vi "set temperature SINEWAVE - V1.vi"(10 "sweep folder path":path, 11 "Set Temperature PID":T1) -> (0 "next set temperature":dbl, 1 "set temperature points":dbl[](array[numeric]), 2 "time points (min)":dbl[](array[numeric]), 3 "Set Temperature PID OUT":T1)   [LabVIEW 2015]
uses:
  Set Temperature PID - Control.ctl
  next chunk read-write PID -- action.ctl
  ctl -- name dispatcher -- action.ctl
  file -- 9w path.vi
  array -- find index - real.vi
  array -- interpolate -- i.vi
  ctl -- name dispatcher.vi
  Q -- check range -- i -- real.vi
  Q - not nan -- real.vi
  <vilib>/Utility/libraryn.llb/Check if File or Folder Exists.vi
  file -- read list of lines.vi
  parse -- find first line.vi
  parse -- get list of matches -- numbers.vi
  <vilib>/Utility/file.llb/Write To Spreadsheet File.vi
  <vilib>/Utility/file.llb/Write To Spreadsheet File (string).vi
  <vilib>/gmath/function.llb/Binomial Coefficient.vi
panel:
  out "time(min)":dbl
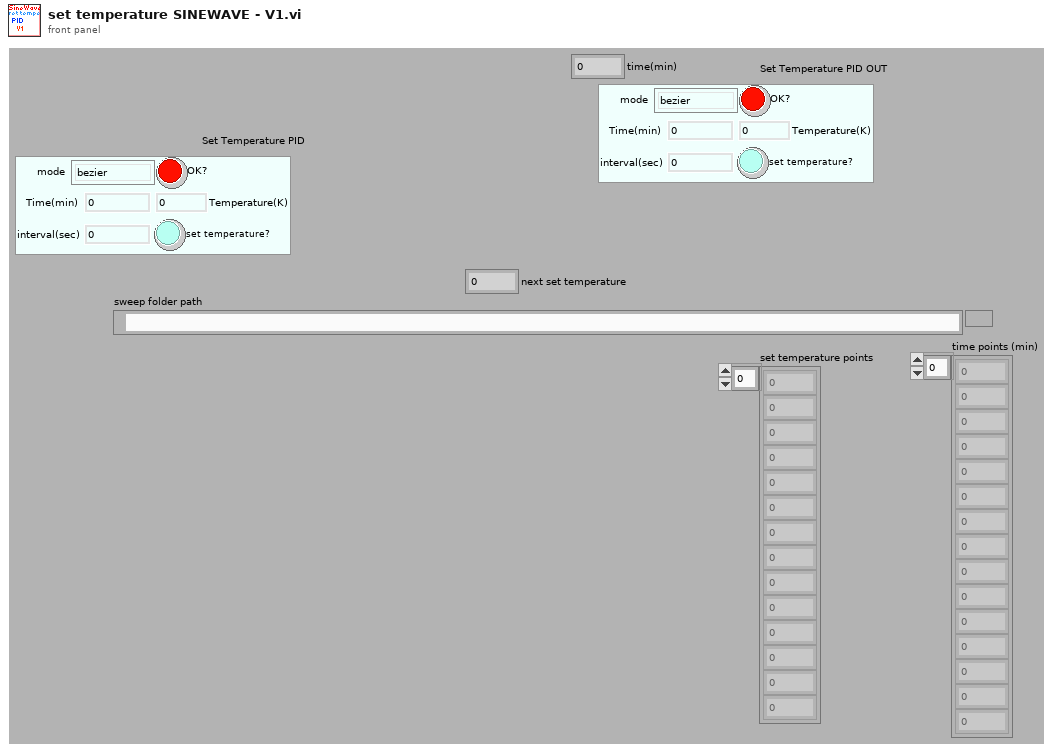
[diagram p1: front panel]
types:
  T1 = typedef "Set Temperature PID - Control.ctl" = cluster{"mode ":enum16{"bezier", "sine wave"}, "set temperature?":bool, "Time(min)":dbl, "Temperature(K)":dbl, "OK?":bool, "interval(sec)":dbl}
  T2 = typedef "next chunk read-write PID -- action.ctl" = enum16{"read", "interpolate", "append col", "write", "write PID col", "append PID col", "interpolate - bezier"}
  T3 = typedef "ctl -- name dispatcher -- action.ctl" = enum16{"peak frequency", "peak frequency DUMP", "peak gamma DUMP", "peak gamma", "peak frequency TEST", "peak gamma TEST", "ultrasonic power", "time in gamma", "set temperature ", "set temperature timer", "peak default gamma", "last scan file", "peak freq gamma TEST", "peak NAMES", "errors", "P_I_D", "P", "I", "D", "power vs time", "power vs time TIMER", "void", "power log", "set temperature - SINE", "itc ltc log", "peak - time in gamma"}
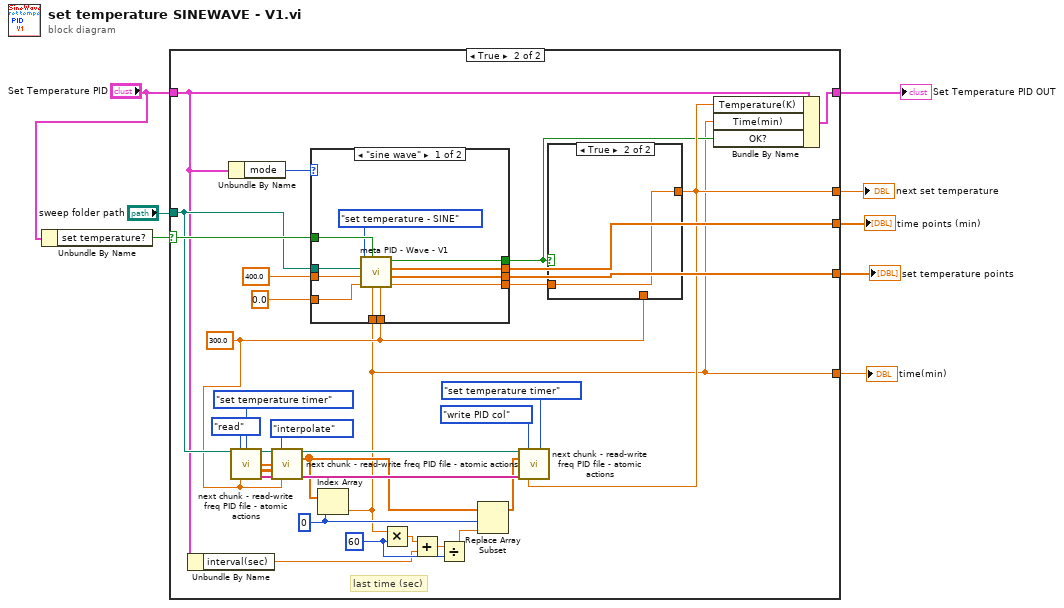
[diagram p0: block diagram]
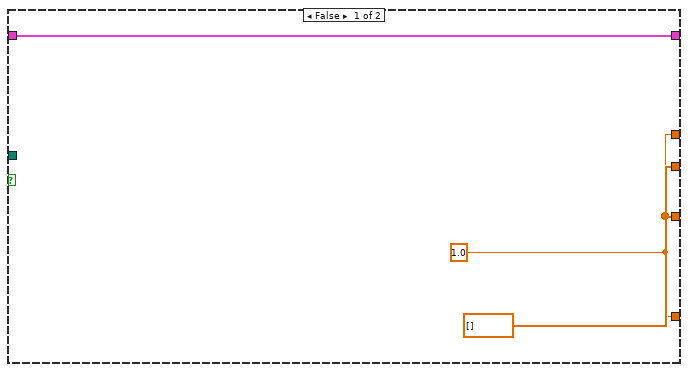
[diagram p2: hidden frame]
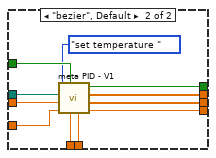
[diagram p3: hidden frame]
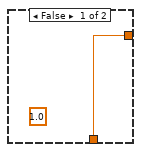
[diagram p4: hidden frame]
diagram:
  n1 = Unbundle By Name("Set Temperature PID") -> ("set temperature?"=w1:bool)
  n2 = case shown="True" w1 {
    selector: w1 -> [_ w41]
    tunnel: "sweep folder path" -> [_ w36]
    tunnel: [w10 w17] -> w7
    tunnel: [w11 w39] -> w6
    tunnel: [w11 w40] -> w5
    tunnel: [w10 w15] -> w4
    tunnel: "Set Temperature PID" -> [w9 w13]
    tunnel: [w9 w14] -> w3
    frame False {
      w11 = dbl[] [] ("temperatures")
      w10 = 1.0 ("upper")
    }
    frame True {
      w19 = 300.0 ("temperature")
      w27 = 0 ("index")
      w22 = 60
      # "last time (sec)"
      n3 = Unbundle By Name(w13) -> ("interval(sec)"=w12:dbl)
      n4 = Unbundle By Name(w13) -> ("mode"=w18:enum16{"bezier", "sine wave"})
      n5 = call "next chunk - read-write freq PID file - atomic actions .vi"("sweep folder path"=w36, "PID action"=next_chunk_read-write_PID_--_action."read", "ctl kind IN"=ctl_--_name_dispatcher_--_action."set temperature timer", "temperature"=w19) -> ("sweep folder path out"=w35:path, "temperatures"=w31:dbl[], "frequencies"=w30:dbl[][], "header"=w32:string[])  [unwired: 7 in, 1 out]
      n6 = call "next chunk - read-write freq PID file - atomic actions .vi"("PID action"=next_chunk_read-write_PID_--_action."interpolate", "temperatures IN"=w31, "frequencies IN"=w30, "header IN"=w32, "temperature"=w19) -> ("PID freq"=w23:dbl[], "header"=w28:string[])  [unwired: 6 in, 3 out]
      n7 = Index Array(array=w23, index=w27) -> (element=w15:dbl)
      n8 = case shown="\"sine wave\"" w18 {
        tunnel: 0.0 ("lower") -> [w54 w65]
        tunnel: 400.0 ("upper") -> [w53 w64]
        tunnel: w41 -> [w52 w63]
        tunnel: [w51 w62] -> w40
        tunnel: [w50 w61] -> w39
        tunnel: [w49 w60] -> w16
        tunnel: w36 -> [w48 w59]
        tunnel: [w47 w58] -> w20
        tunnel: w19 -> [w45 w56]
        tunnel: w15 -> [w44 w55]
        frame "sine wave" {
          n9 = call "meta PID - Wave - V1.vi"("default output"=w45, "input parameter"=w44, "control?"=w52, "lower limit"=w54, "upper limit"=w53, "sweep folder path"=w48, "ctl name dispatch"=ctl_--_name_dispatcher_--_action."set temperature - SINE") -> ("output"=w47:dbl, "frequencies"=w51:dbl[], "temperatures"=w50:dbl[], "ok"=w49:bool)  [unwired: 1 in]
        }
        frame "bezier", Default {
          n10 = call "meta PID - V1.vi"("default output"=w56, "input parameter"=w55, "control?"=w63, "lower limit"=w65, "upper limit"=w64, "sweep folder path"=w59, "ctl name dispatch"=ctl_--_name_dispatcher_--_action."set temperature ") -> ("bezier output"=w58:dbl, "frequencies"=w62:dbl[], "temperatures"=w61:dbl[], "ok"=w60:bool)  [unwired: 1 in]
        }
      }
      n11 = Multiply(x=w15, y=w22) -> (x*y=w21:dbl)
      n12 = Add(x=w21, y=w12) -> (x+y=w25:dbl)
      n13 = Divide(x=w25, y=w22) -> (x/y=w24:dbl)
      n14 = Replace Array Subset(array=w23, new element=w24, index=w27) -> (w26:dbl[])
      n15 = case shown="True" w16 {
        tunnel: [w66 w67] -> w17
        tunnel: w20 -> [_ w67]
        tunnel: w19 -> [w66 _]
        frame False {
          (unwired) 1.0 ("upper")
        }
        frame True {
        }
      }
      n16 = call "next chunk - read-write freq PID file - atomic actions .vi"("sweep folder path"=w35, "PID action"=next_chunk_read-write_PID_--_action."write PID col", "ctl kind OUT"=ctl_--_name_dispatcher_--_action."set temperature timer", "PID freq IN"=w26, "header IN"=w28, "temperature"=w17) -> ()  [unwired: 5 in, 5 out]
      n17 = Bundle By Name(cluster=w13, "Temperature(K)"=w17, "Time(min)"=w15, "OK?"=w16) -> (w14:T1)
    }
  }
  "next set temperature" <- w7
  "time points (min)" <- w6
  "set temperature points" <- w5
  "time(min)" <- w4
  "Set Temperature PID OUT" <- w3
